vi "Boolean Definition.vi"(11 "Boolean in":refnum<class "Boolean.lvclass">) -> (2 "Definition":T1)   [LabVIEW 2020, in "Conditu2.lvlib" / "Columns.lvlib" / "Boolean.lvclass"]
uses:
  Boolean.lvclass
  Definition.ctl
  Boolean.lvclass/Boolean.ctl
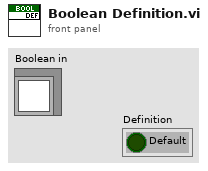
[diagram p1: front panel]
types:
  T1 = typedef "Conditu2.lvlib/Columns.lvlib/Boolean.lvclass/Definition.ctl" = cluster{"Default":bool}
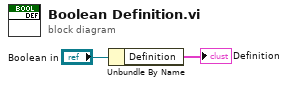
[diagram p0: block diagram]
diagram:
  n1 = Unbundle By Name("Boolean in") -> ("Definition"=→"Definition":T1)
